vi "gradient descent 2.0.vi"(8 "tolerance":dbl=0.001, 9 "weight_smooth":dbl=0.4, 10 "weight_data":dbl=0.6, 11 "Path":dbl[][](array[numeric])) -> (3 "Smooth Path":dbl[][](array[numeric]))   [LabVIEW 2018]
panel:
  out "Graph":cluster{"Array":dbl[], "Array":dbl[]}[](graph)
  out "iterations":i32
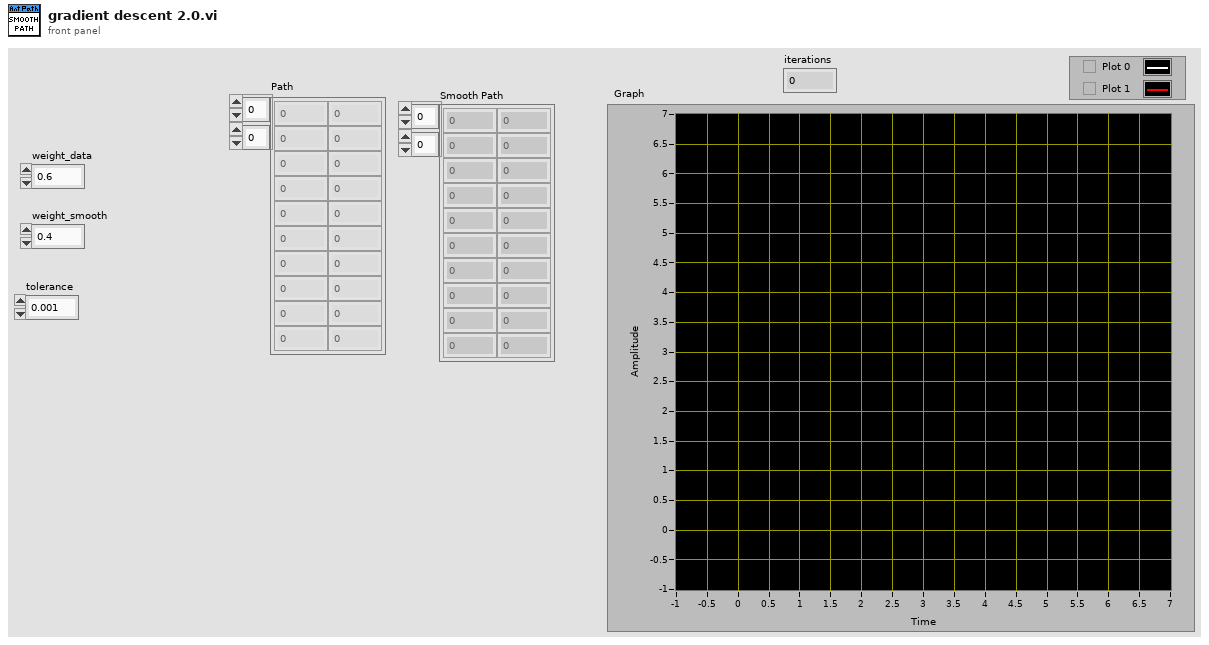
[diagram p1: front panel]
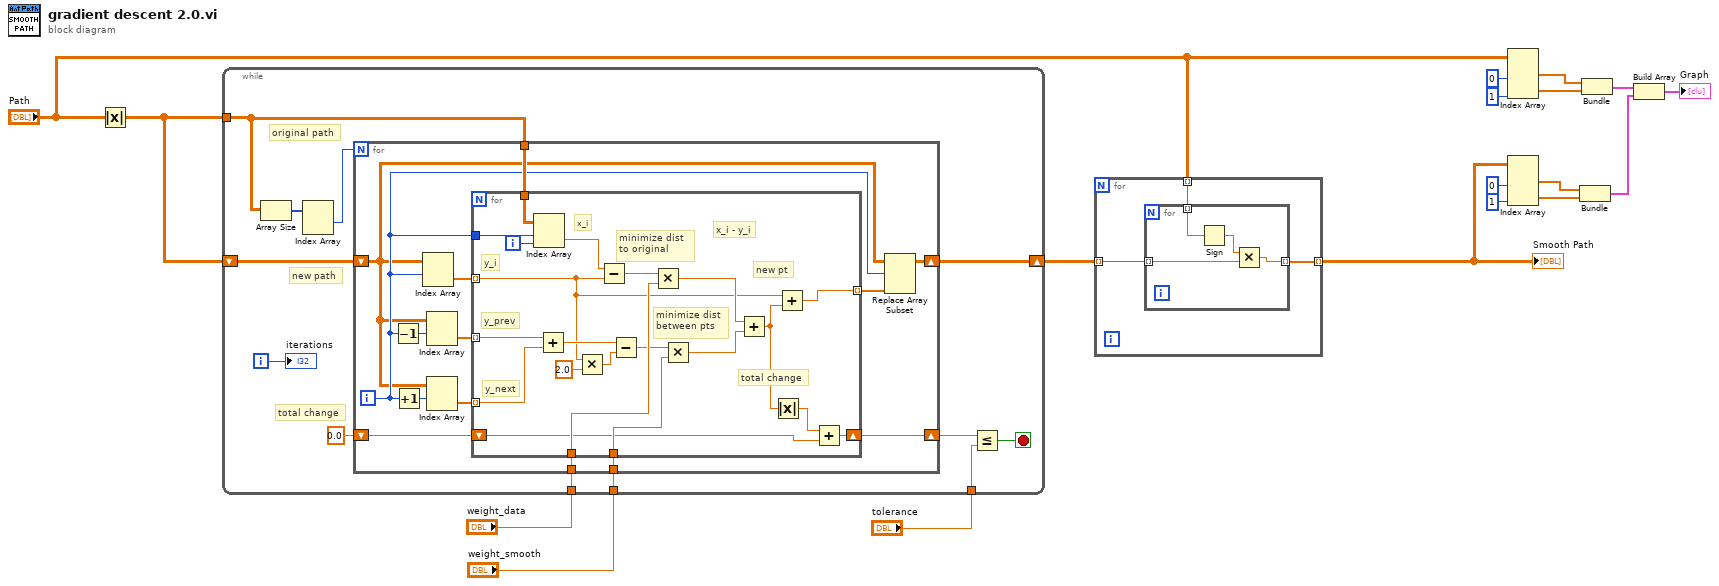
[diagram p0: block diagram]
diagram:
  n1 = Absolute Value(x="Path") -> (abs(x)=w1:dbl[][])
  n2 = while {
    tunnel: w1 -> [w26]
    tunnel: "weight_data" -> [w29]
    tunnel: "weight_smooth" -> [w28]
    shift-right: [w25] -> w4
    shift-left: w1 -> [w27]
    tunnel: "tolerance" -> [w23]
    i -> [w21]
    stop <- w22 stop-if-true
    # "total change"
    # "new path"
    # "original path"
    n3 = Array Size(array=w26) -> (size(s)=w30:i32[])
    n4 = Index Array(array=w30) -> (element #1=w20:i32)  [unwired: 2 in, 1 out]
    n5 = for {
      N: w20 -> [_]
      tunnel: w26 -> [w43]
      tunnel: w29 -> [w38]
      tunnel: w28 -> [w37]
      shift-right: [w31] -> w24
      shift-left: 0.0 -> [w33]
      shift-right: [w34] -> w25
      shift-left: w27 -> [w36]
      i -> [w42]
      n6 = Decrement(x=w42) -> (x-1=w32:i32)
      n7 = Increment(x=w42) -> (x+1=w41:i32)
      n8 = Index Array(array=w36, index (row)=w42) -> (element=w44:dbl[])  [unwired: 1 in]
      n9 = Index Array(array=w36, index (row)=w32) -> (element=w40:dbl[])  [unwired: 1 in]
      n10 = Index Array(array=w36, index (row)=w41) -> (element=w39:dbl[])  [unwired: 1 in]
      n11 = for {
        tunnel: w44 -> [w49] mode=indexing
        tunnel: w43 -> [w65]
        tunnel: w42 -> [w64]
        tunnel: w40 -> [w59] mode=indexing
        tunnel: w39 -> [w58] mode=indexing
        tunnel: w38 -> [w60]
        tunnel: w37 -> [w53]
        tunnel: [w50] -> w35 mode=indexing
        shift-right: [w45] -> w31
        shift-left: w33 -> [w46]
        i -> [w63]
        # "new pt"
        # "total change"
        # "minimize dist\nbetween pts"
        # "minimize dist \nto original"
        # "x_i - y_i"
        # "y_next"
        # "y_prev"
        # "y_i"
        # "x_i"
        n12 = Index Array(array=w65, index (row)=w64, index (col)=w63) -> (element=w62:dbl)
        n13 = Add(x=w59, y=w58) -> (x+y=w56:dbl)
        n14 = Multiply(x=w49, y=2.0) -> (x*y=w55:dbl)
        n15 = Subtract(x=w62, y=w49) -> (x-y=w61:dbl)
        n16 = Subtract(x=w56, y=w55) -> (x-y=w54:dbl)
        n17 = Multiply(x=w61, y=w60) -> (x*y=w52:dbl)
        n18 = Multiply(x=w54, y=w53) -> (x*y=w51:dbl)
        n19 = Add(x=w52, y=w51) -> (x+y=w48:dbl)
        n20 = Absolute Value(x=w48) -> (abs(x)=w47:dbl)
        n21 = Add(x=w49, y=w48) -> (x+y=w50:dbl)
        n22 = Add(x=w47, y=w46) -> (x+y=w45:dbl)
      }
      n23 = Replace Array Subset(array=w36, new element=w35, index (row)=w42) -> (w34:dbl[][])  [unwired: 1 in]
    }
    n24 = Less Or Equal?(x=w24, y=w23) -> (x <= y?=w22:bool)
    "iterations" <- w21
  }
  n25 = for {
    tunnel: w4 -> [w68] mode=indexing
    tunnel: [w67] -> w3 mode=indexing
    tunnel: "Path" -> [w66] mode=indexing
    n26 = for {
      tunnel: w68 -> [w72] mode=indexing
      tunnel: [w71] -> w67 mode=indexing
      tunnel: w66 -> [w69] mode=indexing
      n27 = Sign(1:w69) -> (0:w70:dbl)
      n28 = Multiply(x=w70, y=w72) -> (x*y=w71:dbl)
    }
  }
  "Smooth Path" <- w3
  n29 = Index Array(array="Path", index (col) #1=0 ("disabled index (col)"), index (col) #2=1 ("index (col)")) -> (element #1=w13:dbl[], element #2=w12:dbl[])  [unwired: 2 in]
  n30 = Index Array(array=w3, index (col) #1=0 ("index (col)"), index (col) #2=1 ("index (col)")) -> (element #1=w8:dbl[], element #2=w7:dbl[])  [unwired: 2 in]
  n31 = Bundle(w8, w7) -> (w6:cluster{dbl[], dbl[]})  [unwired: 1 in]
  n32 = Bundle("Path"=w13, "Path"=w12) -> (w11:cluster{"Path":dbl[], "Path":dbl[]})  [unwired: 1 in]
  n33 = Build Array(w11, w6) -> (→"Graph":cluster{"Path":dbl[], "Path":dbl[]}[])
